vi "Create All Message Queues.vi"(8 "error in (no error)":errorcluster) -> (0 "error out":errorcluster, 3 "Message Queues out":T1)   [LabVIEW 2016, in "Message Queue.lvlib"]
doc: "This VI creates and initializes all the message queues for your application. If your application requires more than one message queue, right-click the \"Message Queues\" constant above and select Open Type Def. Add the new Message Queue(s) to the type definition, then initialize them in this VI."
uses:
  Message Queue.lvlib
  All Message Queues.ctl
  Message Cluster.ctl
  Enqueue Message (Single).vi
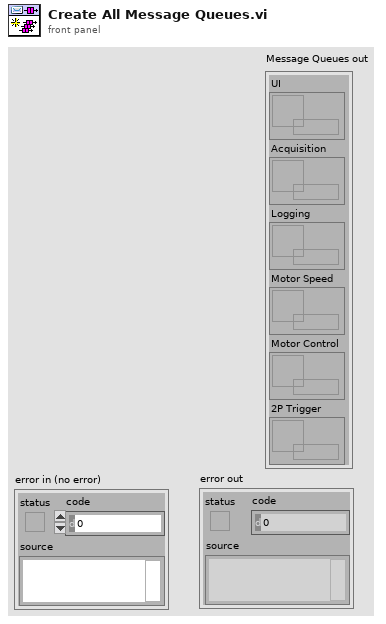
[diagram p1: front panel]
types:
  T1 = typedef "Message Queue.lvlib/All Message Queues.ctl" = cluster{"UI":refnum<queue>, "Acquisition":refnum<queue>, "Logging":refnum<queue>, "Motor Speed":refnum<queue>, "Motor Control":refnum<queue>, "2P Trigger":refnum<queue>}
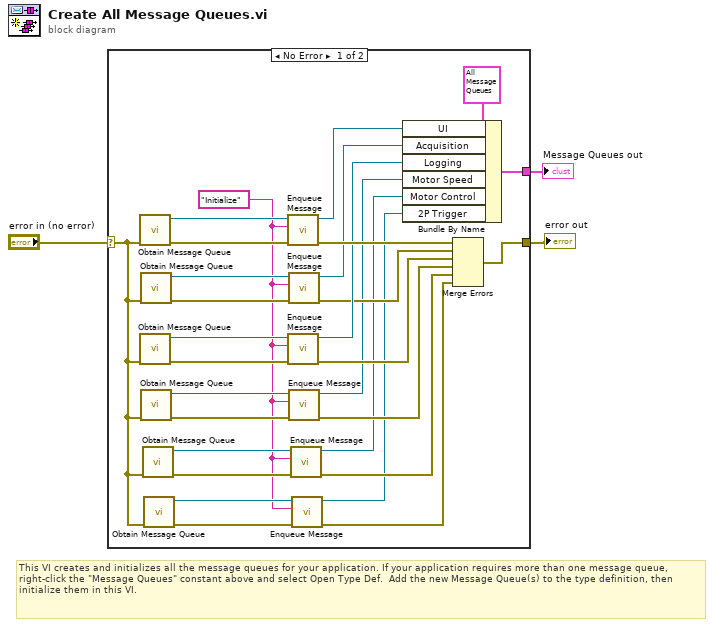
[diagram p0: block diagram]
diagram:
  # "This VI creates and initializes all the message queues for your application. If your application requires more than one message queue, right-click the \"Message Queues\" constant above and select Open Type Def.  Add the new Message Queue(s) to the type definition, then initialize them in this VI."
  n1 = case shown="No Error" "error in (no error)" {
    selector: "error in (no error)" -> [w7 w33]
    tunnel: [w20 w33] -> w3
    tunnel: [w30 _] -> w2
    frame No Error {
      w6 = "Initialize" ("Message")
      n2 = call "Obtain Message Queue.vi"("error in (no error)"=w7) -> ("error out"=w29:errorcluster, "Message Queue"=w28:refnum<queue>)  [unwired: 9 in]
      n3 = call "Obtain Message Queue.vi"("error in (no error)"=w7) -> ("error out"=w25:errorcluster, "Message Queue"=w24:refnum<queue>)  [unwired: 9 in]
      n4 = call "Obtain Message Queue.vi"("error in (no error)"=w7) -> ("error out"=w26:errorcluster, "Message Queue"=w27:refnum<queue>)  [unwired: 9 in]
      n5 = call "Obtain Message Queue.vi"("error in (no error)"=w7) -> ("error out"=w17:errorcluster, "Message Queue"=w16:refnum<queue>)  [unwired: 9 in]
      n6 = call "Obtain Message Queue.vi"("error in (no error)"=w7) -> ("error out"=w12:errorcluster, "Message Queue"=w13:refnum<queue>)  [unwired: 9 in]
      n7 = call "Obtain Message Queue.vi"("error in (no error)"=w7) -> ("error out"=w9:errorcluster, "Message Queue"=w8:refnum<queue>)  [unwired: 9 in]
      n8 = call-poly "Enqueue Message.vi"("error in (no error)"=w29, "Message"=w6, "Message Queue"=w28) -> ("error out"=w32:errorcluster, "dup Message Queue"=w23:refnum<queue>)  [unwired: 7 in]
      n9 = call-poly "Enqueue Message.vi"("error in (no error)"=w25, "Message"=w6, "Message Queue"=w24) -> ("error out"=w18:errorcluster, "dup Message Queue"=w21:refnum<queue>)  [unwired: 7 in]
      n10 = call-poly "Enqueue Message.vi"("error in (no error)"=w26, "Message"=w6, "Message Queue"=w27) -> ("error out"=w19:errorcluster, "dup Message Queue"=w22:refnum<queue>)  [unwired: 7 in]
      n11 = call-poly "Enqueue Message.vi"("error in (no error)"=w17, "Message"=w6, "Message Queue"=w16) -> ("error out"=w15:errorcluster, "dup Message Queue"=w14:refnum<queue>)  [unwired: 7 in]
      n12 = call-poly "Enqueue Message.vi"("error in (no error)"=w12, "Message"=w6, "Message Queue"=w13) -> ("error out"=w10:errorcluster, "dup Message Queue"=w11:refnum<queue>)  [unwired: 7 in]
      n13 = call-poly "Enqueue Message.vi"("error in (no error)"=w9, "Message"=w6, "Message Queue"=w8) -> ("error out"=w5:errorcluster, "dup Message Queue"=w4:refnum<queue>)  [unwired: 7 in]
      n14 = Bundle By Name(cluster=T1 {"UI"=refnum, "Acquisition"=refnum, "Logging"=refnum, "Motor Speed"=refnum, "Motor Control"=refnum, "2P Trigger"=refnum} ("Message Queues"), "UI"=w23, "Acquisition"=w22, "Logging"=w21, "Motor Speed"=w14, "Motor Control"=w11, "2P Trigger"=w4) -> (w30:T1)
      n15 = Merge Errors(w32, w19, w18, w15, w10, w5) -> (w20:errorcluster)
    }
    frame Error {
    }
  }
  "Message Queues out" <- w2
  "error out" <- w3
